vi "LINX - Analog Read N Channels.vi"() -> ()   [LabVIEW 2011, in "LMH-LINX.lvlib"]
doc: "This example demonstrates how to read N channels of analog input from a LINX device."
uses:
  vi.lib/MakerHub/LINX/LMH-LINX.lvlib
  vi.lib/MakerHub/LINX/Public/Peripherals/Analog/Analog Read N Chans.vi
panel:
  in  "AI Channel(s)":u8[](array[numeric])
  in  "Stop Button":bool
  out "Analog Data":T1(graph)
  out "Loop Rate (Hz)":u32
  in  "Serial Port":refnum<visa-resource-name>
  # "Analog Read N Channels Example (Serial Interface)\n\nThis example demonstrates how to read N channels of analog input values from a LINX device connected to the host computer via Serial / USB.\n\nInstructions\n1. Select the COM Port associated with the LINX Device.\n2. Select the Analog Channels to read.\n3. Click the Run Arrow."
  # "LINX Device Settings"
  # "Circuit Schematic"
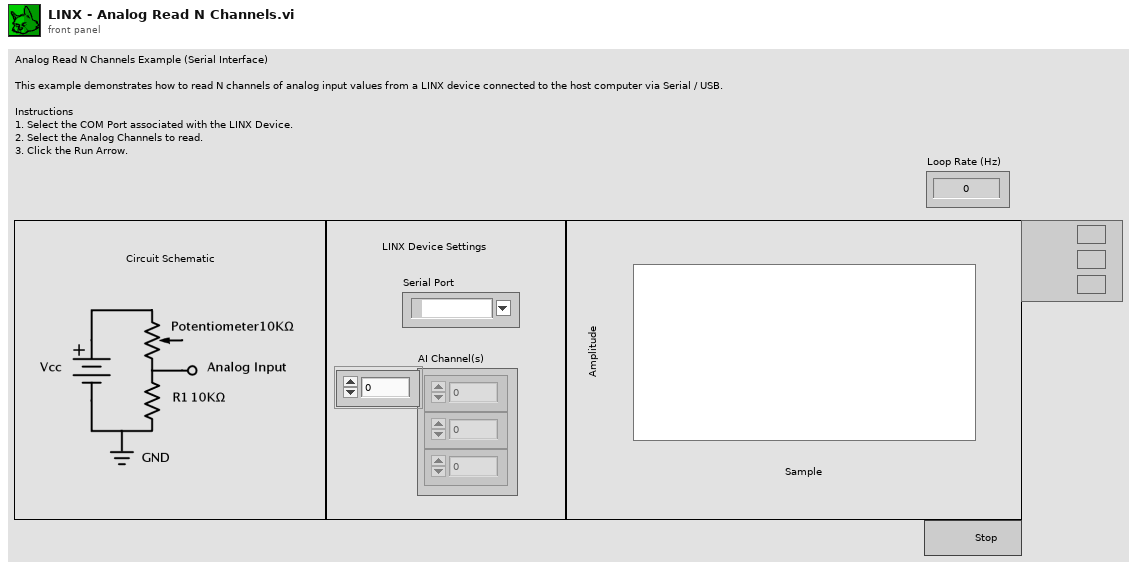
[diagram p1: front panel]
types:
  T1 = cluster{"Voltages[0]":dbl, "Voltages[1]":dbl, "Voltages[2]":dbl, "Voltages[3]":dbl, "Voltages[4]":dbl, "Voltages[5]":dbl, "Voltages[6]":dbl, "Voltages[7]":dbl, "Voltages[8]":dbl}
  T2 = typedef "LMH-LINX.lvlib/LINX Ref.ctl" = cluster{"Platform":T3, "Interface":T4, "LINX Device Config":T5}
  T3 = typedef "LMH-LINX.lvlib/Platform.ctl" = enum16{"LINX", "myRIO"}
  T4 = typedef "LMH-LINX.lvlib/Interface.ctl" = enum16{"Serial", "TCP"}
  T5 = typedef "LMH-LINX.lvlib/Device.lvlib/LINX Device Config.ctl" = cluster{"Interface":T4, "COM Port":refnum<visa-resource-name>, "TCP Configuration":T6, "Device Family":u8, "Device ID":u8, "Device Name":string, "TCP Ref":refnum<k5>, "Channels":T7}
  T6 = typedef "LMH-LINX.lvlib/Device.lvlib/TCP Config.ctl" = cluster{"IP Address":string, "Port":u16}
  T7 = typedef "LMH-LINX.lvlib/Channels.ctl" = cluster{"DI":u8[], "DO":u8[], "AI":u8[], "AO":u8[], "PWM":u8[], "QE":u8[], "UART":u8[], "I2C 2":u8[], "SPI":u8[], "CAN":u8[], "Servo":u8[], "AI Ref (V)":dbl, "AO Ref (V)":dbl, "AO Resolution (Bits)":u8}
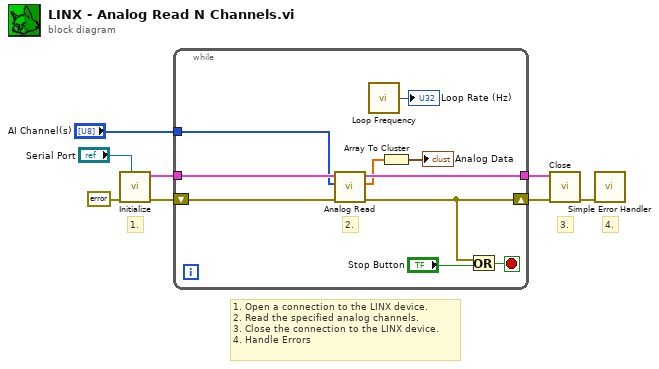
[diagram p0: block diagram]
diagram:
  # "1. Open a connection to the LINX device.\n2. Read the specified analog channels.\n3. Close the connection to the LINX device.\n4. Handle Errors"
  # "4."
  # "3."
  # "1."
  n1 = call "Initialize.vi"("Serial Port"="Serial Port", "Error In"=errorcluster {"status"=FALSE, "code"=0, "source"=""}) -> ("Error Out"=w7:errorcluster, "LINX Ref"=w8:T2)  [unwired: 7 in, 1 out]
  n2 = while {
    tunnel: w8 -> [w18]
    tunnel: [w16] -> w6
    shift-right: [w13] -> w5
    shift-left: w7 -> [w17]
    tunnel: "AI Channel(s)" -> [w11]
    stop <- w15 stop-if-true
    # "2."
    n3 = call-poly "Analog Read.vi"("Error In"=w17, "AI Channel(s)"=w11, "LINX Resource"=w18) -> ("Error Out"=w13:errorcluster, "Voltages"=w10:dbl[], "LINX Resource"=w16:T2)  [unwired: 5 in, 1 out]
    n4 = call "Loop Frequency.vi"() -> ("Loop Rate (Hz)"=→"Loop Rate (Hz)":u32)
    n5 = Array To Cluster(array=w10) -> (cluster=→"Analog Data":T1)
    n6 = Or(x=w13, y="Stop Button") -> (x .or. y?=w15:bool)
  }
  n7 = call "Close.vi"("Error In"=w5, "LINX Resource"=w6) -> ("Error Out"=w3:errorcluster)  [unwired: 8 in, 1 out]
  n8 = call <vilib>:"Simple Error Handler.vi"("error in (no error)"=w3) -> ()  [unwired: 4 in, 5 out]
